vi "simple add.vi"() -> ()   [LabVIEW 2017]
panel:
  out "Boolean":bool
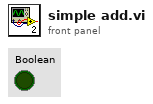
[diagram p1: front panel]
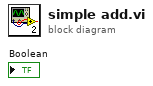
[diagram p0: block diagram]
diagram:
